vi "Run All.vi"(8 "Error In":errorcluster) -> (0 "Error Out":errorcluster)   [LabVIEW 2018, in "Tests.lvlib" / "Render.lvlib"]
uses:
  Render.lvlib
  <vilib>/addons/_JKI Toolkits/Caraya/classes/Test/Test.lvclass
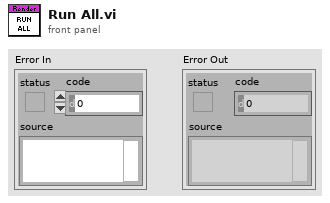
[diagram p1: front panel]
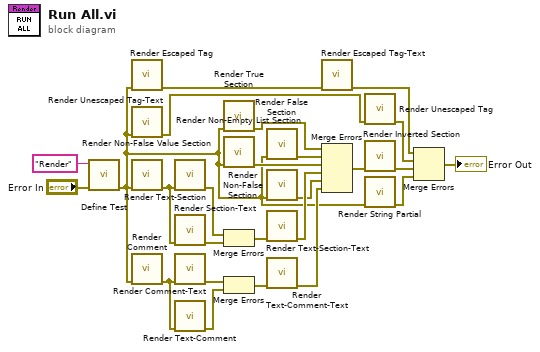
[diagram p0: block diagram]
diagram:
  n1 = call <vilib>:"Define Test.vi"("error in (no error)"="Error In", "Label (VI Title)"="Render") -> ("error out"=w2:errorcluster)  [unwired: 9 in]
  n2 = call "Render Escaped Tag.vi"("Error In"=w2) -> ("Error Out"=w23:errorcluster)  [unwired: 10 in]
  n3 = call "Render Unescaped Tag-Text.vi"("Error In"=w2) -> ("Error Out"=w20:errorcluster)  [unwired: 10 in]
  n4 = call "Render Non-False Value Section.vi"("Error In"=w2) -> ("Error Out"=w5:errorcluster)  [unwired: 10 in]
  n5 = call "Render Comment.vi"("Error In"=w2) -> ("Error Out"=w8:errorcluster)  [unwired: 10 in]
  n6 = call "Render Text-Section.vi"("Error In"=w5) -> ("Error Out"=w18:errorcluster)  [unwired: 10 in]
  n7 = call "Render Section-Text.vi"("Error In"=w5) -> ("Error Out"=w3:errorcluster)  [unwired: 10 in]
  n8 = call "Render Comment-Text.vi"("Error In"=w8) -> ("Error Out"=w10:errorcluster)  [unwired: 10 in]
  n9 = call "Render Text-Comment.vi"("Error In"=w8) -> ("Error Out"=w6:errorcluster)  [unwired: 10 in]
  n10 = call "Render True Section.vi"("Error In"=w2) -> ("Error Out"=w17:errorcluster)  [unwired: 10 in]
  n11 = call "Render Non-Empty List Section.vi"("Error In"=w2) -> ("Error Out"=w15:errorcluster)  [unwired: 10 in]
  n12 = Merge Errors(w18, w3) -> (w4:errorcluster)
  n13 = Merge Errors(w10, w6) -> (w7:errorcluster)
  n14 = call "Render False Section.vi"("Error In"=w2) -> ("Error Out"=w16:errorcluster)  [unwired: 10 in]
  n15 = call "Render Non-False Section.vi"("Error In"=w2) -> ("Error Out"=w13:errorcluster)  [unwired: 10 in]
  n16 = call "Render Text-Section-Text.vi"("Error In"=w4) -> ("Error Out"=w14:errorcluster)  [unwired: 10 in]
  n17 = call "Render Text-Comment-Text.vi"("Error In"=w7) -> ("Error Out"=w9:errorcluster)  [unwired: 10 in]
  n18 = call "Render Escaped Tag-Text.vi"("Error In"=w23) -> ("Error Out"=w22:errorcluster)  [unwired: 10 in]
  n19 = Merge Errors(w17, w16, w15, w14, w13, w9) -> (w12:errorcluster)
  n20 = call "Render Unescaped Tag.vi"("Error In"=w20) -> ("Error Out"=w19:errorcluster)  [unwired: 10 in]
  n21 = call "Render Inverted Section.vi"("Error In"=w12) -> ("Error Out"=w11:errorcluster)  [unwired: 10 in]
  n22 = call "Render String Partial.vi"("Error In"=w2) -> ("Error Out"=w1:errorcluster)  [unwired: 10 in]
  n23 = Merge Errors(w22, w19, w11, w1) -> (→"Error Out":errorcluster)
